vi "correction-left-15(SubVI).vi"   [LabVIEW 2016]
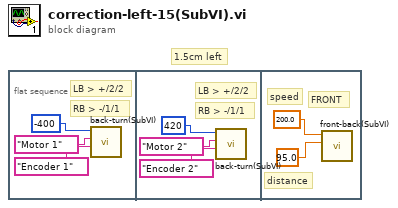
[diagram p0: block diagram]
diagram:
  # "1.5cm left"
  n1 = flat-sequence {
    frame #0 {
      # "RB > -/1/1"
      # "LB > +/2/2"
      n2 = call "back-turn(SubVI).vi"("Select Encoder"="Encoder 1", "Select Channel"="Motor 1", "Motor Encoder Target"=-400) -> ()  [unwired: 9 in]
    }
    frame #1 {
      # "RB > -/1/1"
      # "LB > +/2/2"
      n3 = call "back-turn(SubVI).vi"("Select Encoder"="Encoder 2", "Select Channel"="Motor 2", "Motor Encoder Target"=420) -> ()  [unwired: 9 in]
    }
    frame #2 {
      # "speed"
      # "distance"
      # "FRONT"
      n4 = call "front-back(SubVI).vi"("distance"=95.0, "speed"=200.0) -> ()  [unwired: 10 in]
    }
  }
